vi "Dialog Load Settings.vi"(8 "Error In":errorcluster, 10 "Title Bar String":string, 11 "Settings IN":T1[](array[typedef])) -> (0 "Error Out":errorcluster, 3 "Cancelled?":bool)   [LabVIEW 2012]
doc: "SciScan 1.2 160622"
uses:
  Custom Controls and Typedefs/GFG Variable for IO.ctl
  Dialog Load Settings_UI Refnums.ctl
  CommonResource VIs/Timing/Timer Commands.ctl
panel:
  in  "Select/Un-select All":bool=TRUE
  in  "Selection Array":bool[](array[boolean])
  in  "Parameters (To be Modified)":i32(listbox)
  out "Comments":string
  out "New Value":variant
  out "Current Value":variant
  in  "Cancel Button":bool
  in  "OK Button":bool
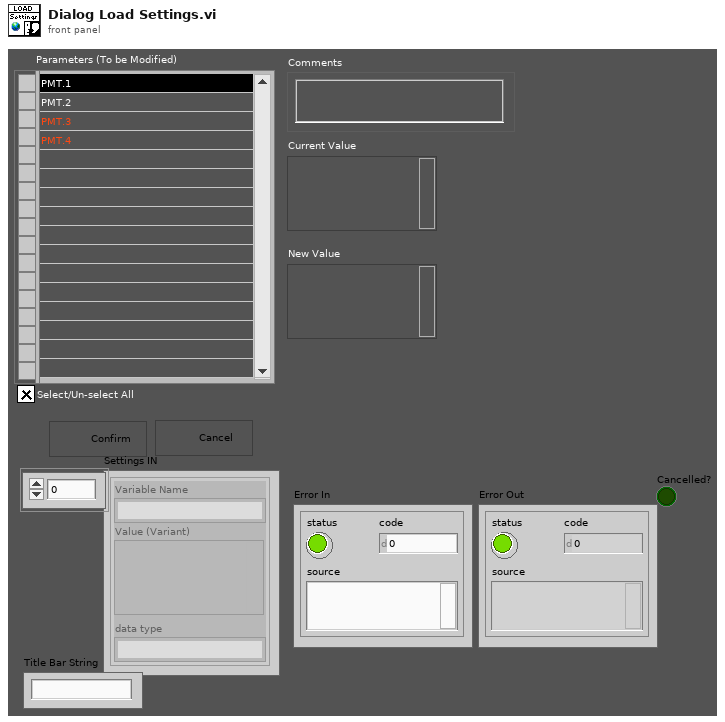
[diagram p1: front panel]
types:
  T1 = typedef "GFG Variable for IO.ctl" = cluster{"Variable Name":string, "Value (Variant)":variant, "data type":string}
  T2 = enum16{"Select Item", "Deselect Item", "Select All", "Deselect All"}
  T3 = typedef "Dialog Load Settings_UI Refnums.ctl" = cluster{"Params":refnum<vi>, "Selection Arr":refnum<vi>, "Curr. Val":refnum<vi>, "New. Val":refnum<vi>, "Comments":refnum<vi>, "Select ALL":refnum<vi>}
  T4 = typedef "Timer Commands.ctl" = enum16{"Clear All", "Start", "Pause", "Check Time"}
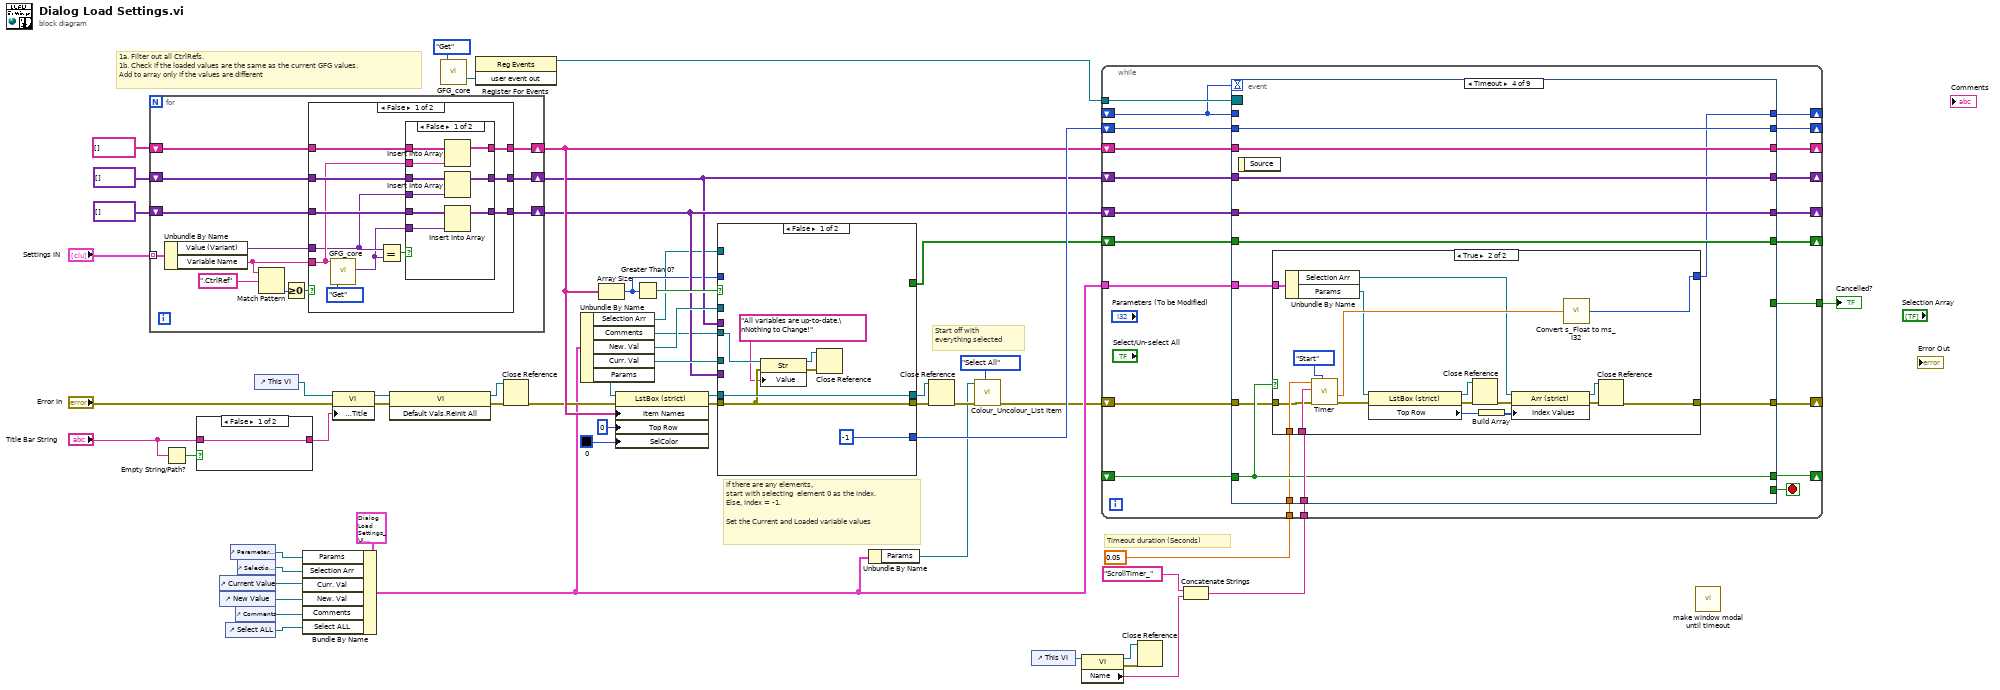
[diagram p0: block diagram]
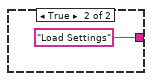
[diagram p2: hidden frame]
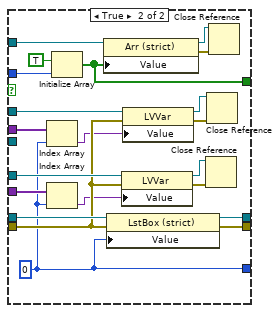
[diagram p3: hidden frame]
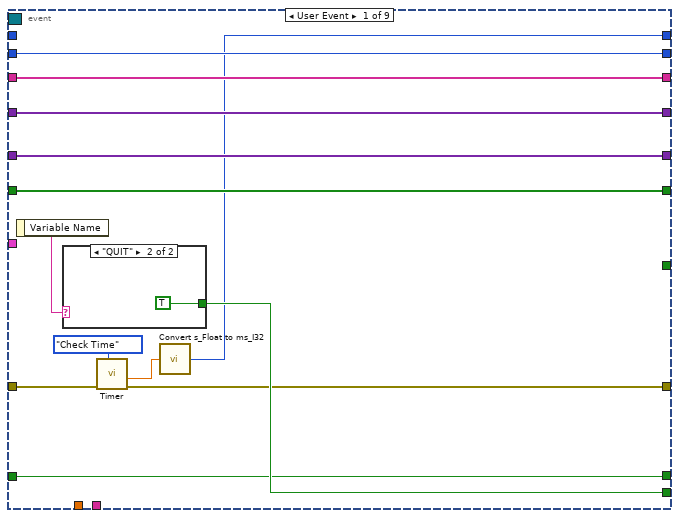
[diagram p6: hidden frame]
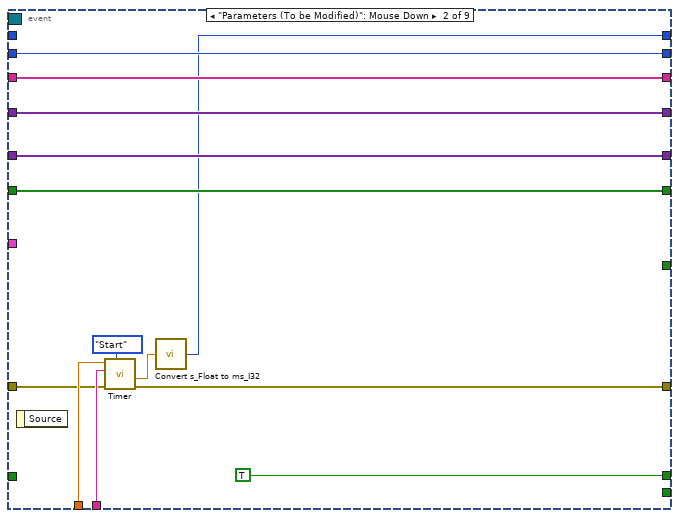
[diagram p8: hidden frame]
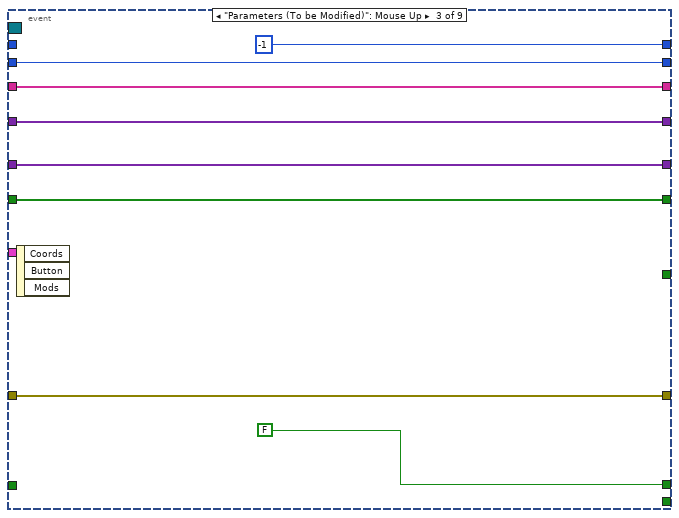
[diagram p9: hidden frame]
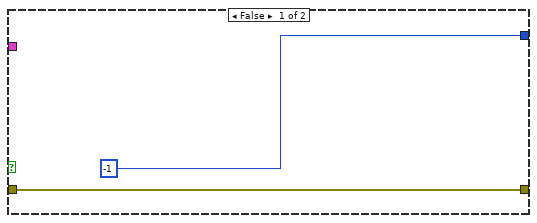
[diagram p10: hidden frame]
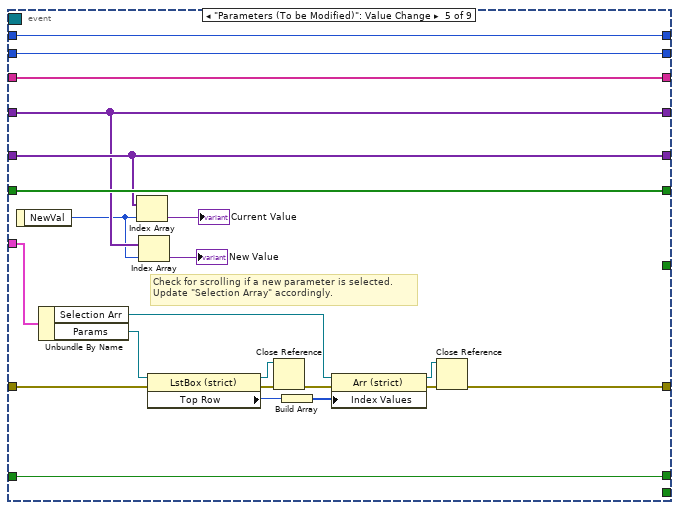
[diagram p11: hidden frame]
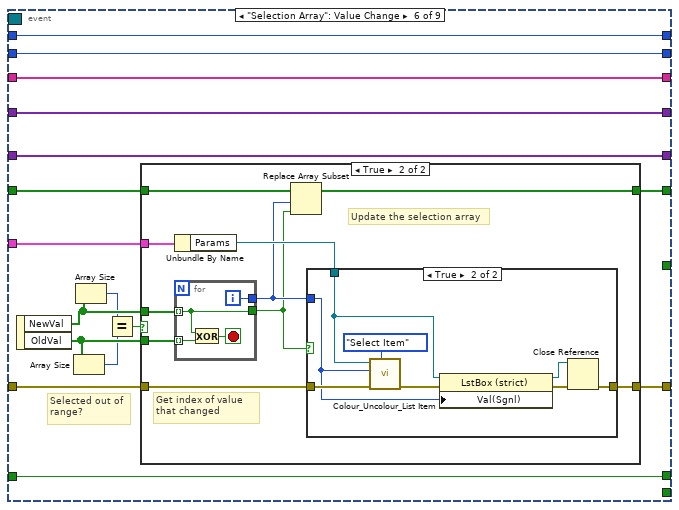
[diagram p12: hidden frame]
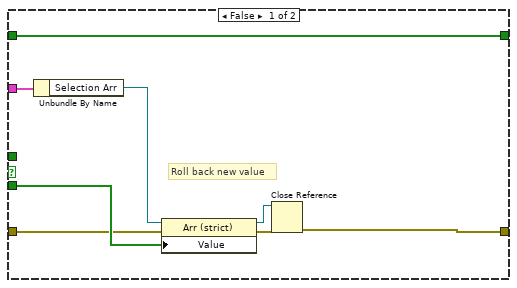
[diagram p13: hidden frame]
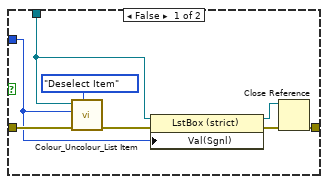
[diagram p14: hidden frame]
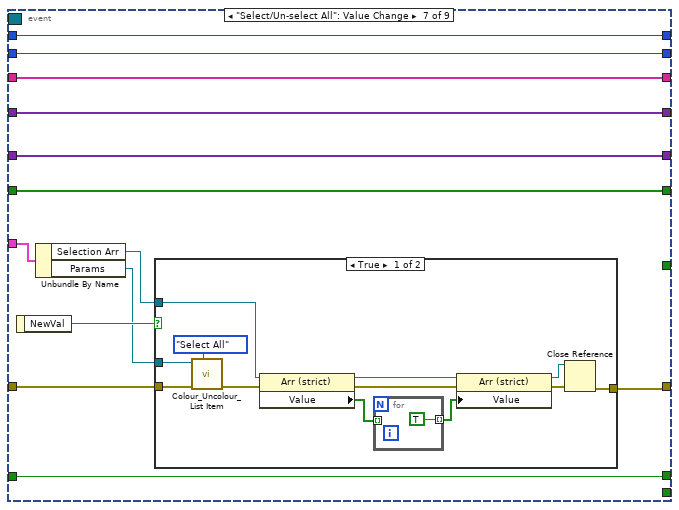
[diagram p15: hidden frame]
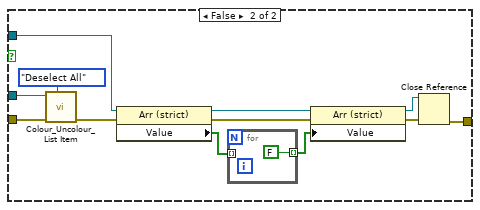
[diagram p16: hidden frame]
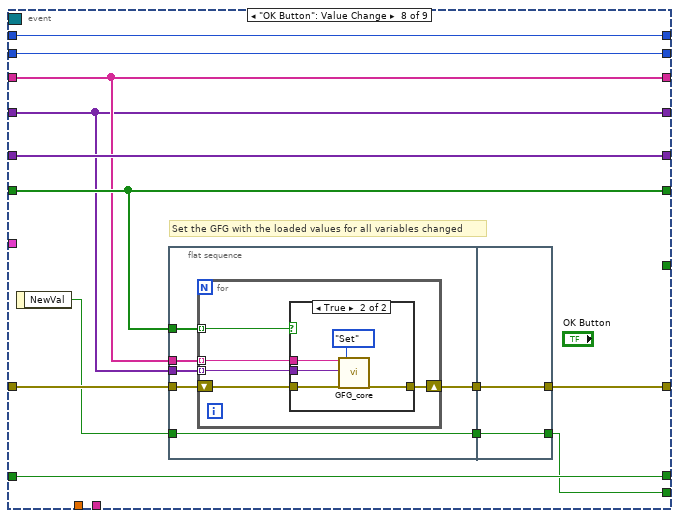
[diagram p17: hidden frame]
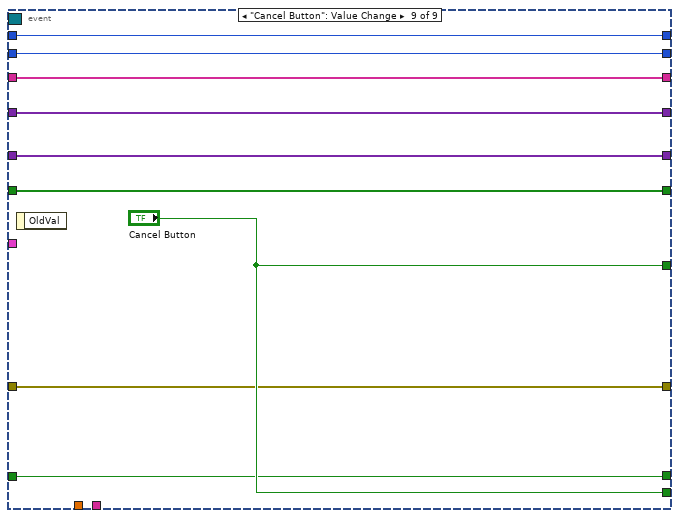
[diagram p19: hidden frame]
diagram:
  # "Start off with everything selected"
  # "Timeout duration (Seconds)"
  # "If there are any elements,\nstart with selecting  element 0 as the index. Else, index = -1.\n\nSet the Current and Loaded variable values"
  # "1a. Filter out all CtrlRefs.\n1b. Check if the loaded values are the same as the current GFG values.\nAdd to array only if the values are different"
  n1 = for {
    tunnel: "Settings IN" -> [w67] mode=indexing
    shift-right: [w61] -> w31
    shift-left: string[] [] -> [w60]
    shift-right: [w59] -> w29
    shift-left: variant[] [] -> [w58]
    shift-right: [w57] -> w30
    shift-left: variant[] [] -> [w56]
    n2 = Unbundle By Name(w67) -> ("Value (Variant)"=w63:variant, "Variable Name"=w62:string)
    n3 = Match Pattern(string=w62, regular expression=".CtrlRef") -> (offset past match=w65:i32)  [unwired: 1 in, 3 out]
    n4 = Greater Or Equal To 0?(x=w65) -> (x >= 0?=w64:bool)
    n5 = case shown="False" w64 {
      tunnel: w63 -> [w69 _]
      tunnel: w62 -> [w70 _]
      tunnel: [w76 w93] -> w61
      tunnel: w60 -> [w75 w93]
      tunnel: [w74 w92] -> w59
      tunnel: w58 -> [w73 w92]
      tunnel: [w72 w91] -> w57
      tunnel: w56 -> [w71 w91]
      frame False {
        n6 = call "GFG_core.vi"("Variable Name in"=w70, "Action"=enum16{"Init", "Set", "Get", "Clear"}."Get") -> ("Variant Out"=w68:variant)  [unwired: 11 in, 6 out]
        n7 = Equal?(x=w69, y=w68) -> (x = y?=w77:bool)
        n8 = case shown="False" w77 {
          tunnel: [w85 w90] -> w76
          tunnel: w75 -> [w87 w90]
          tunnel: [w83 w89] -> w74
          tunnel: w73 -> [w84 w89]
          tunnel: [w79 w88] -> w72
          tunnel: w71 -> [w81 w88]
          tunnel: w70 -> [w86 _]
          tunnel: w69 -> [w82 _]
          tunnel: w68 -> [w80 _]
          frame False {
            n9 = Insert Into Array(array=w87, new element=w86) -> (w85:string[])  [unwired: 1 in]
            n10 = Insert Into Array(array=w84, new element=w82) -> (w83:variant[])  [unwired: 1 in]
            n11 = Insert Into Array(array=w81, new element=w80) -> (w79:variant[])  [unwired: 1 in]
          }
          frame True {
          }
        }
      }
      frame True {
        # "It is a control ref.\n --Ignore!"
      }
    }
  }
  n12 = Empty String/Path?(string/path="Title Bar String") -> (empty?=w9:bool)
  n13 = case shown="False" w9 {
    tunnel: "Title Bar String" -> [w94 _]
    tunnel: [w94 "Load Settings" ("Title Bar String")] -> w7
    frame False {
    }
    frame True {
    }
  }
  n14 = control-ref of="Current Value"() -> (w46:refnum<vi>)
  n15 = control-ref of="New Value"() -> (w45:refnum<vi>)
  n16 = control-ref of="Select ALL"() -> (w24:refnum<vi>)
  n17 = control-ref of="Parameters (To be Modified)"() -> (w48:refnum<vi>)
  n18 = control-ref of="Comments"() -> (w44:refnum<vi>)
  n19 = control-ref of="Selection Array"() -> (w47:refnum<vi>)
  n20 = control-ref of="This VI"() -> (w14:refnum<vi>)
  n21 = Bundle By Name(cluster=T3 {"Params"=refnum, "Selection Arr"=refnum, "Curr. Val"=refnum, "New. Val"=refnum, "Comments"=refnum, "Select ALL"=refnum} ("Dialog Load Settings_UI Refnums"), "Params"=w48, "Selection Arr"=w47, "Curr. Val"=w46, "New. Val"=w45, "Comments"=w44, "Select ALL"=w24) -> (w17:T3)
  n22 = property class="VI"(reference=w14, error in="Error In", "Front Panel.Title"=w7) -> (reference out=w12:refnum<vi>, error out=w13:errorcluster)
  n23 = invoke class="VI" method="Default Vals.Reinit All"(reference=w12, error in=w13) -> (reference out=w26:refnum<vi>, error out=w27:errorcluster)  [unwired: 1 in, 1 out]
  n24 = call "GFG_core.vi"("Action"=enum16{"Init", "Set", "Get", "Clear"}."Get") -> ("user event out"=w55:refnum<user-event>)  [unwired: 12 in, 6 out]
  n25 = register-events(w55) -> (reference out=w54:refnum<event-registration>)  [unwired: 2 in, 1 out]
  n26 = Close Reference(reference=w26, error in (no error)=w27) -> (error out=w25:errorcluster)
  n27 = Unbundle By Name(w17) -> ("Selection Arr"=w22:refnum<vi>, "Comments"=w28:refnum<vi>, "New. Val"=w32:refnum<vi>, "Curr. Val"=w33:refnum<vi>, "Params"=w43:refnum<vi>)
  n28 = Array Size(array=w31) -> (size(s)=w23:i32)
  n29 = property class="LstBox (strict)"(reference=w43, error in=w25, "Item Names"=w31, "Top Row"=0, "SelColor"=u32 0) -> (reference out=w39:refnum<vi>, error out=w40:errorcluster)
  n30 = Greater Than 0?(x=w23) -> (x > 0?=w41:bool)
  n31 = case shown="False" w41 {
    tunnel: w40 -> [w99 w118]
    tunnel: w39 -> [w102 w123]
    tunnel: [w99 w122] -> w38
    tunnel: [w102 w121] -> w37
    tunnel: [-1 ("Value") w115] -> w36
    tunnel: w33 -> [_ w120]
    tunnel: w32 -> [_ w119]
    tunnel: w30 -> [_ w117]
    tunnel: w29 -> [_ w116]
    tunnel: w28 -> [w100 _]
    tunnel: w23 -> [_ w108]
    tunnel: w22 -> [_ w106]
    tunnel: [_ w103] -> w21
    frame False {
      n32 = property class="Str"(reference=w100, error in=w99, "Value"="All variables are up-to-date.\nNothing to Change!") -> (reference out=w96:refnum<vi>, error out=w97:errorcluster)
      n33 = Close Reference(reference=w96, error in (no error)=w97) -> ()  [unwired: 1 out]
    }
    frame True {
      w115 = 0 ("Value")
      n34 = Index Array(array=w116, index=w115) -> (element=w114:variant)
      n35 = Index Array(array=w117, index=w115) -> (element=w113:variant)
      n36 = Initialize Array(TRUE, w108) -> (w103:bool[])
      n37 = property class="Arr (strict)"(reference=w106, "Value"=w103) -> (reference out=w104:refnum<vi>, error out=w105:errorcluster)  [unwired: 1 in]
      n38 = property class="LstBox (strict)"(reference=w123, error in=w118, "Value"=w115) -> (reference out=w121:refnum<vi>, error out=w122:errorcluster)
      n39 = property class="LVVar"(reference=w120, error in=w118, "Value"=w113) -> (reference out=w109:refnum<vi>, error out=w110:errorcluster)
      n40 = property class="LVVar"(reference=w119, error in=w118, "Value"=w114) -> (reference out=w111:refnum<vi>, error out=w112:errorcluster)
      n41 = Close Reference(reference=w109, error in (no error)=w110) -> ()  [unwired: 1 out]
      n42 = Close Reference(reference=w111, error in (no error)=w112) -> ()  [unwired: 1 out]
      n43 = Close Reference(reference=w104, error in (no error)=w105) -> ()  [unwired: 1 out]
    }
  }
  n44 = Unbundle By Name(w17) -> ("Params"=w16:refnum<vi>)
  n45 = Close Reference(reference=w37, error in (no error)=w38) -> (error out=w18:errorcluster)
  n46 = call "Colour_Uncolour_List Item.vi"("Enum"=T2."Select All", "Error In"=w18, "LstBox Refnum"=w16) -> ("Error Out"=w15:errorcluster)  [unwired: 8 in]
  n47 = control-ref of="This VI"() -> (w6:refnum<vi>)
  n48 = property class="VI"(reference=w6) -> (reference out=w3:refnum<vi>, error out=w4:errorcluster, "Name"=w2:string)  [unwired: 1 in]
  n49 = Close Reference(reference=w3, error in (no error)=w4) -> ()  [unwired: 1 out]
  n50 = Concatenate Strings("ScrollTimer_", w2) -> (w1:string)
  n51 = while {
    tunnel: w54 -> [w145]
    tunnel: [w143] -> w35
    shift-right: [w141] -> _
    shift-left: w36 -> [w142]
    shift-right: [w134] -> _
    shift-left: w30 -> [w140]
    shift-right: [w135] -> _
    shift-left: w29 -> [w139]
    shift-right: [w136] -> _
    shift-left: w31 -> [w137]
    shift-right: [w133] -> _
    shift-left: w21 -> [w138]
    shift-right: [w132] -> _
    shift-left: _ -> [w131]
    shift-right: [w130] -> _
    shift-left: _ -> [w129]
    tunnel: w1 -> [w128]
    tunnel: 0.05 ("Set Time IN (s)") -> [w127]
    shift-right: [w125] -> _
    shift-left: w15 -> [w126]
    tunnel: w17 -> [w124]
    stop <- w144 stop-if-true
    n52 = event shown="[3] Timeout" {
      selector: w145 -> [_ _ _ _ _ _ _ _ _]
      dyn-events: _ -> [_ _ _ _ _ _ _ _ _]
      timeout: w129 -> [_ _ _ _ _ _ _ _ _]
      tunnel: [w157 _ _ _ _ _ _ w329 "Cancel Button"] -> w144
      tunnel: [_ _ _ _ _ _ _ _ "Cancel Button"] -> w143
      tunnel: w142 -> [w156 w172 w180 w192 w234 w250 w301 w340 w367]
      tunnel: [w156 w172 w180 w192 w234 w250 w301 w340 w367] -> w141
      tunnel: w140 -> [w153 w169 w177 w189 w217 w247 w298 w339 w364]
      tunnel: w139 -> [w154 w170 w178 w190 w216 w248 w299 w333 w365]
      tunnel: w138 -> [w152 w168 w176 w188 w232 w236 w297 w335 w363]
      tunnel: w137 -> [w155 w171 w179 w191 w233 w249 w300 w334 w366]
      tunnel: [w155 w171 w179 w191 w233 w249 w300 w334 w366] -> w136
      tunnel: [w154 w170 w178 w190 w216 w248 w299 w333 w365] -> w135
      tunnel: [w153 w169 w177 w189 w217 w247 w298 w339 w364] -> w134
      tunnel: [w152 w168 w176 w188 w232 w235 w297 w335 w363] -> w133
      tunnel: [w147 TRUE FALSE w186 w229 w246 w296 w337 w360] -> w132
      tunnel: w131 -> [w147 _ _ w186 w229 w246 w296 w337 w360]
      tunnel: [w148 w161 -1 ("milliseconds OUT (I32)") w184 w228 w245 w295 w338 w361] -> w130
      tunnel: w129 -> [_ _ _ _ w228 w245 w295 w338 w361]
      tunnel: w128 -> [_ w164 _ w187 _ _ _ _ _]
      tunnel: w127 -> [_ w165 _ w185 _ _ _ _ _]
      tunnel: w126 -> [w149 w163 w175 w183 w230 w243 w293 w336 w362]
      tunnel: [w146 w160 w175 w181 w227 w242 w289 w332 w362] -> w125
      tunnel: w124 -> [_ _ _ w182 w231 w244 w292 _ _]
      event User Event {
        n53 = event-data() -> ("Variable Name"=w158:string)  [unwired: 1 in]
        n54 = case shown="\"QUIT\"" w158 {
          tunnel: [_ TRUE] -> w157
          frame Default {
          }
          frame "QUIT" {
          }
        }
        n55 = call "Timer.vi"("Timer Command"=Timer_Commands."Check Time", "Error In"=w149) -> ("Error Out"=w146:errorcluster, "Remaining Time (s)"=w150:dbl)  [unwired: 4 in, 4 out]
        n56 = call "Convert s_Float to ms_I32.vi"("Seconds IN (Float)"=w150) -> ("milliseconds OUT (I32)"=w148:i32)
      }
      event "Parameters (To be Modified)": Mouse Down {
        n57 = event-data() -> ()  [unwired: 1 in, 1 out]
        n58 = call "Timer.vi"("Timer Command"=Timer_Commands."Start", "Error In"=w163, "VI name (Optional)"=w164, "Set Time IN (s)"=w165) -> ("Error Out"=w160:errorcluster, "Remaining Time (s)"=w162:dbl)  [unwired: 2 in, 4 out]
        n59 = call "Convert s_Float to ms_I32.vi"("Seconds IN (Float)"=w162) -> ("milliseconds OUT (I32)"=w161:i32)
      }
      event "Parameters (To be Modified)": Mouse Up {
        n60 = event-data() -> ()  [unwired: 1 in, 3 out]
      }
      event Timeout {
        n61 = event-data() -> ()  [unwired: 1 in, 1 out]
        n62 = case shown="True" w186 {
          tunnel: w187 -> [_ w212]
          tunnel: w185 -> [_ w211]
          tunnel: [-1 ("milliseconds OUT (I32)") w208] -> w184
          tunnel: w183 -> [w193 w198]
          tunnel: w182 -> [_ w196]
          tunnel: [w193 w195] -> w181
          frame False {
          }
          frame True {
            n63 = Unbundle By Name(w196) -> ("Selection Arr"=w200:refnum<vi>, "Params"=w199:refnum<vi>)
            n64 = call "Timer.vi"("Timer Command"=Timer_Commands."Start", "Error In"=w198, "VI name (Optional)"=w212, "Set Time IN (s)"=w211) -> ("Error Out"=w197:errorcluster, "Remaining Time (s)"=w209:dbl)  [unwired: 2 in, 4 out]
            n65 = property class="LstBox (strict)"(reference=w199, error in=w197) -> (reference out=w202:refnum<vi>, error out=w201:errorcluster, "Top Row"=w203:i32)
            n66 = Close Reference(reference=w202, error in (no error)=w201) -> (error out=w207:errorcluster)
            n67 = Build Array(w203) -> (w204:i32[])
            n68 = property class="Arr (strict)"(reference=w200, error in=w207, "Index Values"=w204) -> (reference out=w206:refnum<vi>, error out=w205:errorcluster)
            n69 = call "Convert s_Float to ms_I32.vi"("Seconds IN (Float)"=w209) -> ("milliseconds OUT (I32)"=w208:i32)
            n70 = Close Reference(reference=w206, error in (no error)=w205) -> (error out=w195:errorcluster)
          }
        }
      }
      event "Parameters (To be Modified)": Value Change {
        # "Check for scrolling if a new parameter is selected. \nUpdate \"Selection Array\" accordingly."
        n71 = event-data() -> ("NewVal"=w215:i32)  [unwired: 1 in]
        n72 = Unbundle By Name(w231) -> ("Selection Arr"=w219:refnum<vi>, "Params"=w218:refnum<vi>)
        n73 = Index Array(array=w217, index=w215) -> (element=→"Current Value":variant)
        n74 = Index Array(array=w216, index=w215) -> (element=→"New Value":variant)
        n75 = property class="LstBox (strict)"(reference=w218, error in=w230) -> (reference out=w221:refnum<vi>, error out=w220:errorcluster, "Top Row"=w222:i32)
        n76 = Close Reference(reference=w221, error in (no error)=w220) -> (error out=w226:errorcluster)
        n77 = Build Array(w222) -> (w223:i32[])
        n78 = property class="Arr (strict)"(reference=w219, error in=w226, "Index Values"=w223) -> (reference out=w225:refnum<vi>, error out=w224:errorcluster)
        n79 = Close Reference(reference=w225, error in (no error)=w224) -> (error out=w227:errorcluster)
      }
      event "Selection Array": Value Change {
        # "Selected out of\nrange?"
        n80 = event-data() -> ("NewVal"=w241:bool[], "OldVal"=w240:bool[])  [unwired: 1 in]
        n81 = Array Size(array=w240) -> (size(s)=w238:i32)
        n82 = Array Size(array=w241) -> (size(s)=w239:i32)
        n83 = Equal?(x=w239, y=w238) -> (x = y?=w237:bool)
        n84 = case shown="True" w237 {
          tunnel: w244 -> [w258 w268]
          tunnel: w243 -> [w255 w267]
          tunnel: [w252 w265] -> w242
          tunnel: w241 -> [_ w264]
          tunnel: w240 -> [w256 w263]
          tunnel: w236 -> [w251 w262]
          tunnel: [w251 w259] -> w235
          frame False {
            # "Roll back new value"
            n85 = Unbundle By Name(w258) -> ("Selection Arr"=w257:refnum<vi>)
            n86 = property class="Arr (strict)"(reference=w257, error in=w255, "Value"=w256) -> (reference out=w253:refnum<vi>, error out=w254:errorcluster)
            n87 = Close Reference(reference=w253, error in (no error)=w254) -> (error out=w252:errorcluster)
          }
          frame True {
            # "Update the selection array"
            # "Get index of value that changed"
            n88 = Unbundle By Name(w268) -> ("Params"=w266:refnum<vi>)
            n89 = for {
              tunnel: w264 -> [w285] mode=indexing
              tunnel: w263 -> [w288] mode=indexing
              tunnel: [w286] -> w261
              tunnel: [w285] -> w260
              i -> [w286]
              stop <- w287 stop-if-true
              n90 = Exclusive Or(1:w288, 2:w285) -> (0:w287:bool)
            }
            n91 = Replace Array Subset(array=w262, new element=w260, index=w261) -> (w259:bool[])
            n92 = case shown="True" w260 {
              tunnel: w267 -> [w275 w283]
              tunnel: w261 -> [w272 w280]
              tunnel: w266 -> [w274 w282]
              tunnel: [w269 w277] -> w265
              frame False {
                n93 = call "Colour_Uncolour_List Item.vi"("Enum"=T2."Deselect Item", "Error In"=w275, "Index"=w272, "LstBox Refnum"=w274) -> ("Error Out"=w273:errorcluster)  [unwired: 7 in]
                n94 = property class="LstBox (strict)"(reference=w274, error in=w273, "Val(Sgnl)"=w272) -> (reference out=w270:refnum<vi>, error out=w271:errorcluster)
                n95 = Close Reference(reference=w270, error in (no error)=w271) -> (error out=w269:errorcluster)
              }
              frame True {
                n96 = call "Colour_Uncolour_List Item.vi"("Enum"=T2."Select Item", "Error In"=w283, "Index"=w280, "LstBox Refnum"=w282) -> ("Error Out"=w281:errorcluster)  [unwired: 7 in]
                n97 = property class="LstBox (strict)"(reference=w282, error in=w281, "Val(Sgnl)"=w280) -> (reference out=w278:refnum<vi>, error out=w279:errorcluster)
                n98 = Close Reference(reference=w278, error in (no error)=w279) -> (error out=w277:errorcluster)
              }
            }
          }
        }
      }
      event "Select/Un-select All": Value Change {
        n99 = event-data() -> ("NewVal"=w294:bool)  [unwired: 1 in]
        n100 = Unbundle By Name(w292) -> ("Selection Arr"=w290:refnum<vi>, "Params"=w291:refnum<vi>)
        n101 = case shown="True" w294 {
          tunnel: w293 -> [w313 w326]
          tunnel: w291 -> [w311 w324]
          tunnel: w290 -> [w310 w323]
          tunnel: [w302 w315] -> w289
          frame True {
            n102 = call "Colour_Uncolour_List Item.vi"("Enum"=T2."Select All", "Error In"=w313, "LstBox Refnum"=w311) -> ("Error Out"=w309:errorcluster)  [unwired: 8 in]
            n103 = property class="Arr (strict)"(reference=w310, error in=w309) -> (reference out=w307:refnum<vi>, error out=w306:errorcluster, "Value"=w308:bool[])
            n104 = for {
              tunnel: w308 -> [_] mode=indexing
              tunnel: [TRUE] -> w305 mode=indexing
            }
            n105 = property class="Arr (strict)"(reference=w307, error in=w306, "Value"=w305) -> (reference out=w303:refnum<vi>, error out=w304:errorcluster)
            n106 = Close Reference(reference=w303, error in (no error)=w304) -> (error out=w302:errorcluster)
          }
          frame False {
            n107 = call "Colour_Uncolour_List Item.vi"("Enum"=T2."Deselect All", "Error In"=w326, "LstBox Refnum"=w324) -> ("Error Out"=w322:errorcluster)  [unwired: 8 in]
            n108 = property class="Arr (strict)"(reference=w323, error in=w322) -> (reference out=w320:refnum<vi>, error out=w319:errorcluster, "Value"=w321:bool[])
            n109 = for {
              tunnel: w321 -> [_] mode=indexing
              tunnel: [FALSE] -> w318 mode=indexing
            }
            n110 = property class="Arr (strict)"(reference=w320, error in=w319, "Value"=w318) -> (reference out=w316:refnum<vi>, error out=w317:errorcluster)
            n111 = Close Reference(reference=w316, error in (no error)=w317) -> (error out=w315:errorcluster)
          }
        }
      }
      event "OK Button": Value Change {
        # "Set the GFG with the loaded values for all variables changed"
        n112 = event-data() -> ("NewVal"=w330:bool)  [unwired: 1 in]
        n113 = flat-sequence {
          tunnel: w336 -> [w346]
          tunnel: w335 -> [w345]
          tunnel: w334 -> [w344]
          tunnel: w333 -> [w343]
          tunnel: [w342] -> w331
          tunnel: w330 -> [w341]
          tunnel: [w341] -> w328
          tunnel: [w359] -> w332
          tunnel: w331 -> [w359]
          tunnel: [w358] -> w329
          tunnel: w328 -> [w358]
          frame #0 {
            n114 = for {
              shift-right: [w347] -> w342
              shift-left: w346 -> [w348]
              tunnel: w345 -> [w351] mode=indexing
              tunnel: w344 -> [w349] mode=indexing
              tunnel: w343 -> [w350] mode=indexing
              n115 = case shown="True" w351 {
                tunnel: w350 -> [_ w356]
                tunnel: w349 -> [_ w355]
                tunnel: w348 -> [w352 w354]
                tunnel: [w352 w353] -> w347
                frame False {
                }
                frame True {
                  n116 = call "GFG_core.vi"("Variable Name in"=w355, "Variant in"=w356, "error in (no error)"=w354, "Action"=enum16{"Init", "Set", "Get", "Clear"}."Set") -> ("error out"=w353:errorcluster)  [unwired: 9 in, 6 out]
                }
              }
            }
          }
          frame #1 {
          }
        }
      }
      event "Cancel Button": Value Change {
        n117 = event-data() -> ()  [unwired: 1 in, 1 out]
      }
    }
  }
  "Cancelled?" <- w35
  n118 = call "make window modal until timeout.vi"() -> ()  [unwired: 12 in]
